vi "Scope Read 20.vi"(8 "error in (no error)":errorcluster, 9 "Sample Rate":dbl, 10 "Maximum Record Length":dbl, 11 "VISA Refnum in":refnum<visa-resource-name>) -> (0 "error out":errorcluster, 3 "Division Number":i32)   [LabVIEW 2021]
uses:
  <instrlib>/Tektronix MSO5X Series/Tektronix MSO5X Series.lvlib
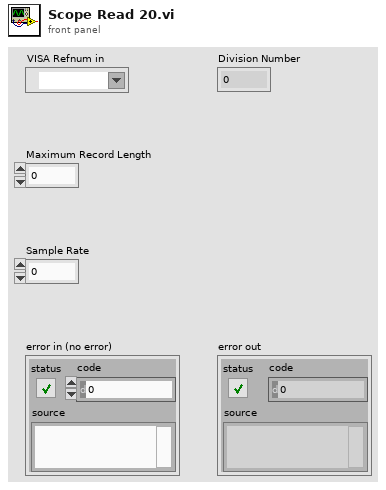
[diagram p1: front panel]
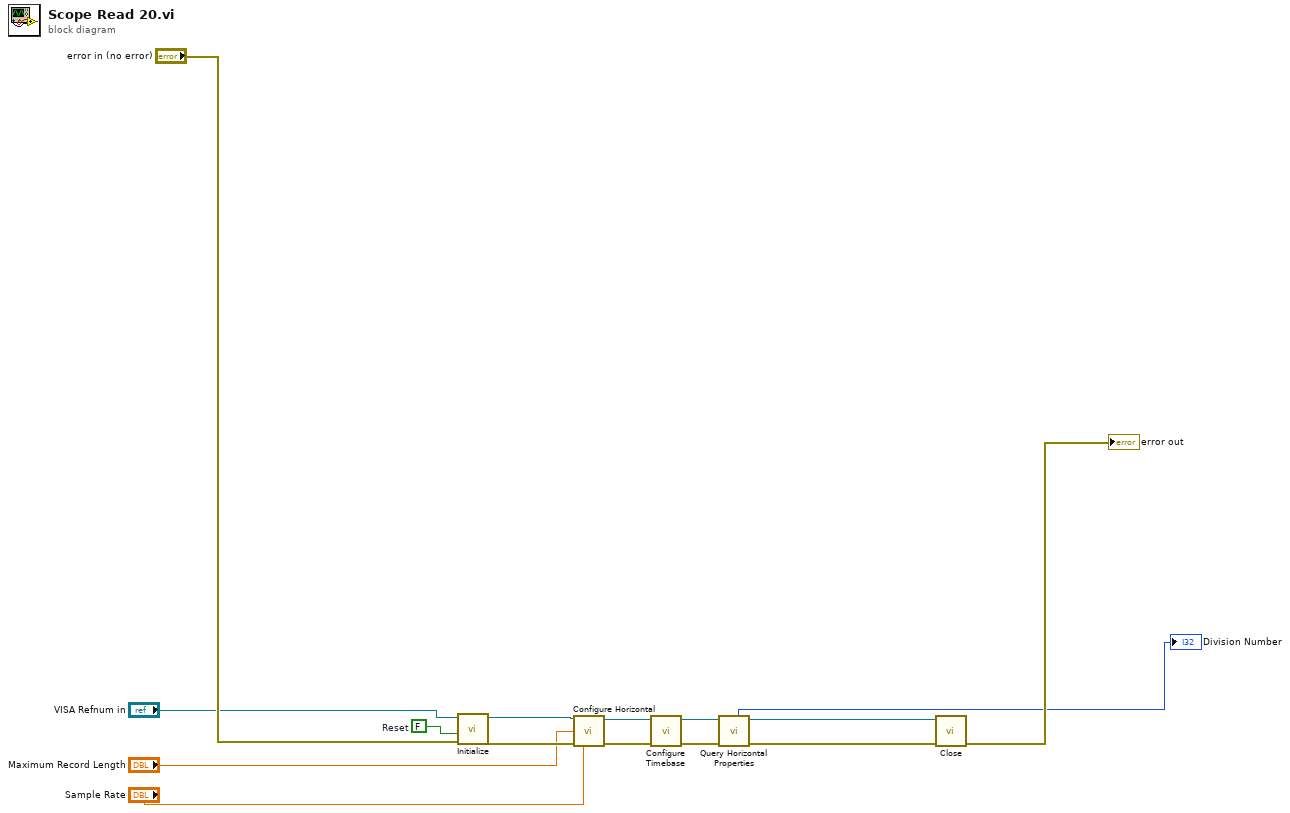
[diagram p0: block diagram]
diagram:
  w12 = FALSE  # Reset
  n1 = call <instrlib>:"Initialize.vi"("error in (no error)"="error in (no error)", "Reset (True)"=w12, "VISA resource name"="VISA Refnum in") -> ("error out"=w10:errorcluster, "VISA resource name out"=w11:refnum<visa-resource-name>)  [unwired: 7 in]
  n2 = call <instrlib>:"Configure Horizontal.vi"("VISA resource name"=w11, "Maximum Record Length (2.5E+8)"="Maximum Record Length", "error in (no error)"=w10, "Sample Rate (3.125E+9)"="Sample Rate") -> ("VISA resource name out"=w4:refnum<visa-resource-name>, "error out"=w3:errorcluster)  [unwired: 10 in]
  n3 = call <instrlib>:"Configure Timebase.vi"("error in (no error)"=w3, "VISA resource name"=w4) -> ("error out"=w2:errorcluster, "VISA resource name out"=w1:refnum<visa-resource-name>)  [unwired: 8 in]
  n4 = call <instrlib>:"Query Horizontal Properties.vi"("error in (no error)"=w2, "VISA resource name"=w1) -> ("error out"=w5:errorcluster, "VISA resource name out"=w6:refnum<visa-resource-name>, "Division Number"=→"Division Number":i32)  [unwired: 5 in, 2 out]
  n5 = call <instrlib>:"Close.vi"("error in (no error)"=w5, "VISA resource name"=w6) -> ("error out"=→"error out":errorcluster)  [unwired: 9 in]
